vi "Send to CS.vi"(8 "error in (no error)":errorcluster, 10 "String to write":string, 11 "CS Emulation in":refnum<class "CS Emulation.lvclass">) -> (0 "error out":errorcluster, 3 "CS Emulation out":refnum<class "CS Emulation.lvclass">)   [LabVIEW 2013, in "CS Emulation.lvclass"]
uses:
  Lib.llb/CS Emulation.lvclass
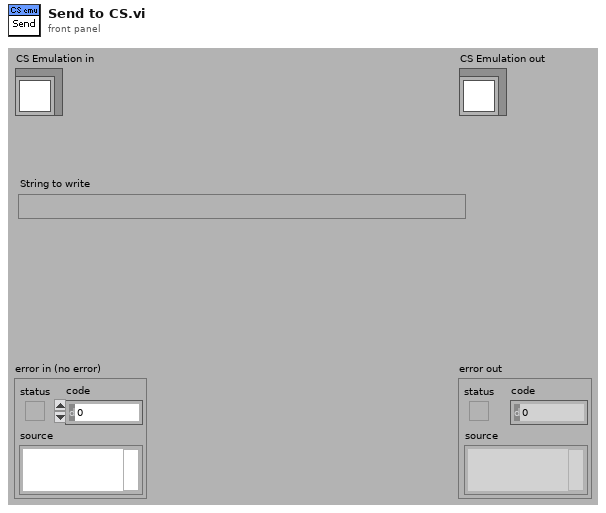
[diagram p1: front panel]
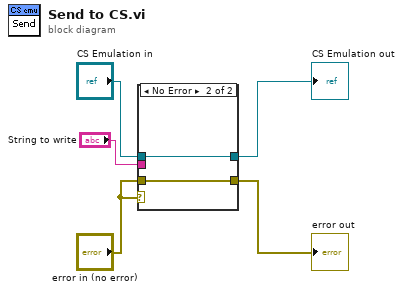
[diagram p0: block diagram]
diagram:
  n1 = case shown="No Error" "error in (no error)" {
    tunnel: [w6 w8] -> w5
    tunnel: [w7 w9] -> w4
    tunnel: "error in (no error)" -> [w6 w8]
    tunnel: "String to write" -> [_ _]
    tunnel: "CS Emulation in" -> [w7 w9]
    frame Error {
    }
    frame No Error {
    }
  }
  "error out" <- w5
  "CS Emulation out" <- w4
